vi "SLM_Holo to BMP.vi"(1 "path to BMP file":path=path "C:/Users/science/Desktop/Filippo The 2nd/LabVIEW/Holos/SLMA/HG_2_2.bmp", 2 "Holo":u32[][](array[numeric])) -> ()   [LabVIEW 2024]
uses:
  <vilib>/Utility/miscctls.llb/LVBoundsTypeDef.ctl
panel:
  in  "Array":u32[](array[numeric])=[1, 2, 3, 4, 5, 6, 7, 8, 9, 10, 11, 12, 13, 14, 15, 16, 17, 18, 19, 20, 21, 22, 23, 24, 25, 26, 27, 28, 29, 30, 31, 32, 33, 34, 35, 36, 37, 38, 39, 40, 41, 42, 43, 44, 45, 46, 47, 48, 49, 50, 51, 52, 53, 54, 55, 56, 57, 58, 59, 60, 61, 62, 63, 64, 65, 66, 67, 68, 69, 70, 71, 72, 73, 74, 75, 76, 77, 78, 79, 80, 81, 82, 83, 84, 85, 86, 87, 88, 89, 90, 91, 92, 93, 94, 95, 96, 97, 98, 99, 100, 101, 102, 103, 104, 105, 106, 107, 108, 109, 110, 111, 112, 113, 114, 115, 116, 117, 118, 119, 120, 121, 122, 123, 124, 125, 126, 127, 128, 129, 130, 131, 132, 133, 134, 135, 136, 137, 138, 139, 140, 141, 142, 143, 144, 145, 146, 147, 148, 149, 150, 151, 152, 153, 154, 155, 156, 157, 158, 159, 160, 161, 162, 163, 164, 165, 166, 167, 168, 169, 170, 171, 172, 173, 174, 175, 176, 177, 178, 179, 180, 181, 182, 183, 184, 185, 186, 187, 188, 189, 190, 191, 192, 193, 194, 195, 196, 197, 198, 199, 200, 201, 202, 203, 204, 205, 206, 207, 208, 209, 210, 211, 212, 213, 214, 215, 216, 217, 218, 219, 220, 221, 222, 223, 224, 225, 226, 227, 228, 229, 230, 231, 232, 233, 234, 235, 236, 237, 238, 239, 240, 241, 242, 243, 244, 245, 246, 247, 248, 249, 250, 251, 252, 253, 254, 255, 256]
  out "holo A":picture
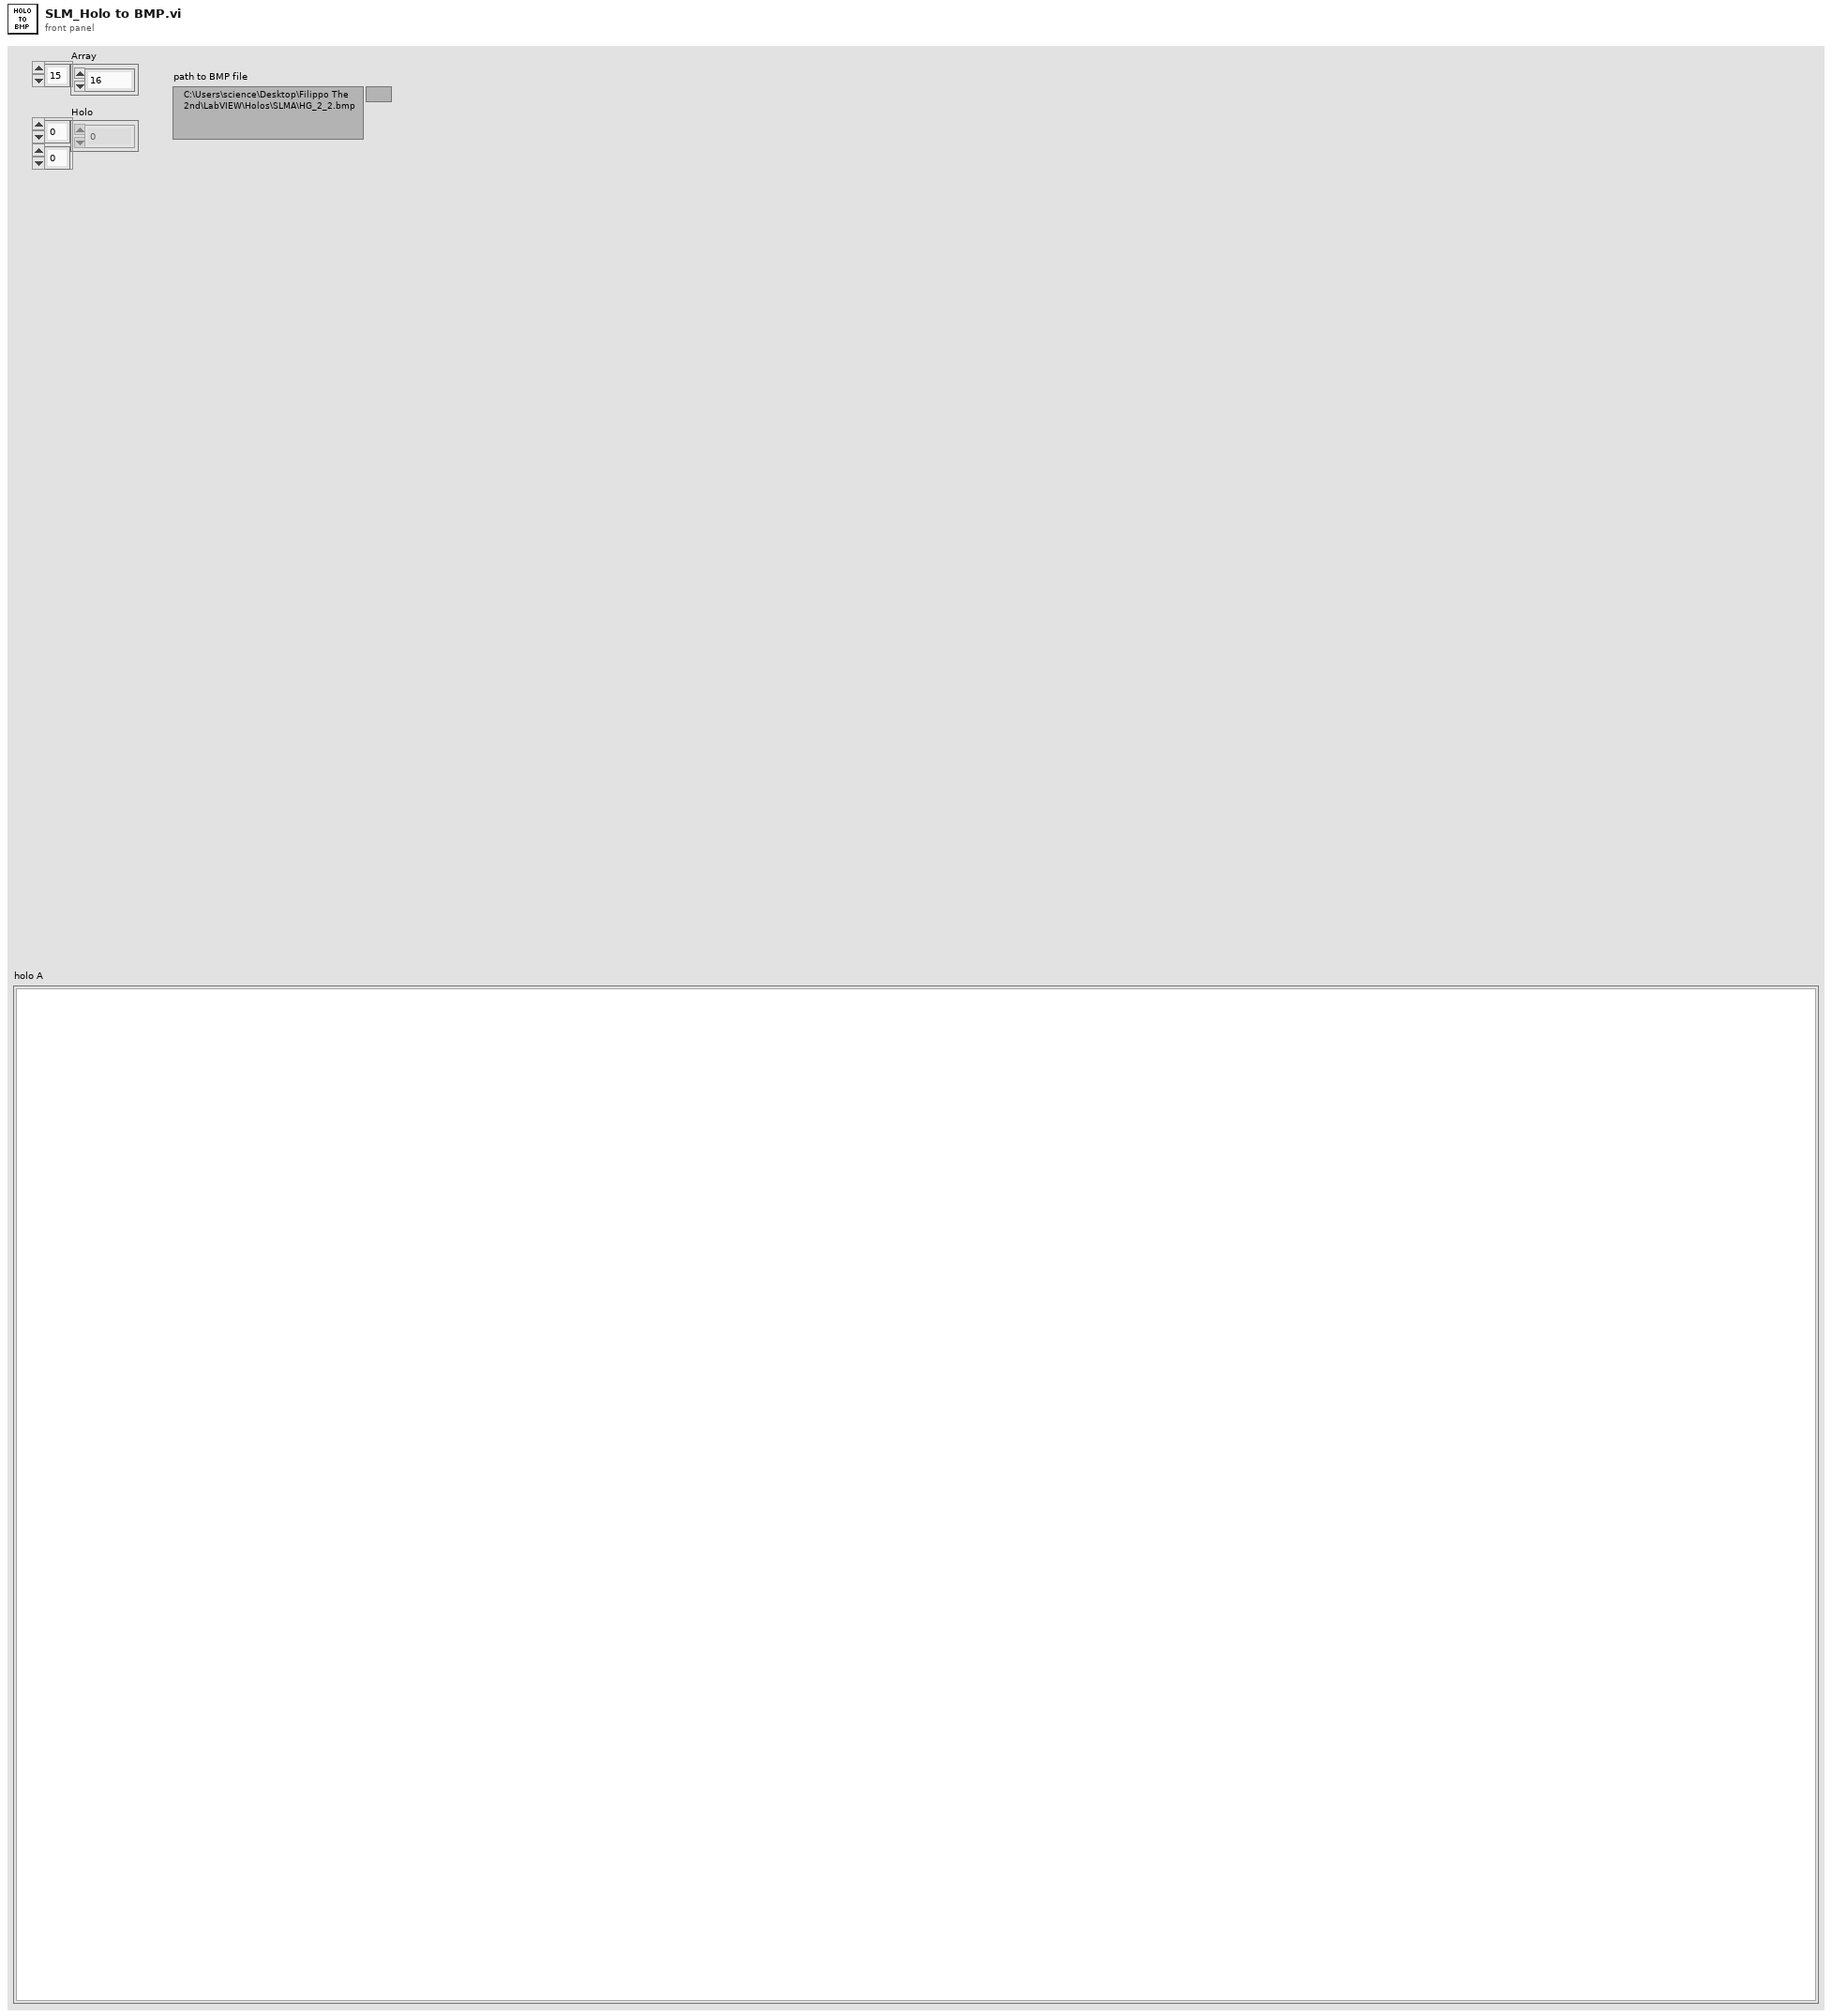
[diagram p1: front panel]
types:
  T1 = typedef "LVBoundsTypeDef.ctl" = cluster{"Width":u32, "Height":u32}
  T2 = cluster{"left":i16, "top":i16, "right":i16, "bottom":i16}
  T3 = typedef "imagedata.ctl" = cluster{"image type":i32, "image depth":i32, "image":u8[], "mask":u8[], "colors":u32[], "Rectangle":cluster{"left":i16, "top":i16, "right":i16, "bottom":i16}}
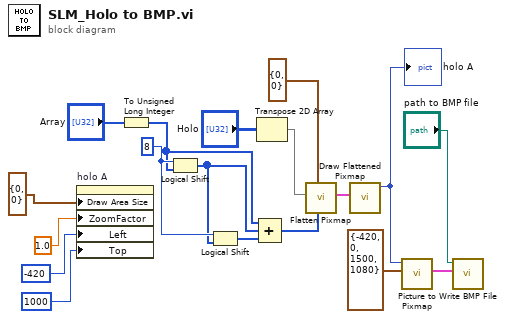
[diagram p0: block diagram]
diagram:
  w15 = i16 8 ("y")
  n1 = property on="holo A" class="Pict"("Draw Area Size"=T1 {"Width"=0, "Height"=0}, "ZoomFactor"=sgl 1.0 ("Zoom Factor"), "Left"=i16 -420 ("Origin:Left"), "Top"=1000 ("Position:Top")) -> ()  [unwired: 2 in, 2 out]
  n2 = To Unsigned Long Integer(number="Array") -> (unsigned 32bit integer=w14:u32[])
  n3 = Logical Shift(y=w15, x=w14) -> (x << y=w13:u32[])
  n4 = Logical Shift(y=w15, x=w13) -> (x << y=w16:u32[])
  n5 = Transpose 2D Array(2D array="Holo") -> (transposed array=w9:u32[][])
  n6 = Compound Arithmetic op=ADD(w14, w13, w16) -> (w12:u32[])
  n7 = call <vilib>:"Flatten Pixmap.vi"("colors"=w12, "top left"=cluster{"x":i16, "y":i16} {"x"=0, "y"=0}, "8-bit pixmap"=w9) -> ("image data"=w11:T3)  [unwired: 8 in]
  n8 = call <vilib>:"Draw Flattened Pixmap.vi"("image data"=w11) -> ("new picture"=w7:picture)  [unwired: 8 in]
  "holo A" <- w7
  n9 = call <vilib>:"Picture to Pixmap.vi"("rect"=T2 {"left"=-420, "top"=0, "right"=1500, "bottom"=1080}, "picture"=w7) -> ("image data"=w6:T3)  [unwired: 8 in, 1 out]
  n10 = call <vilib>:"Write BMP File.vi"("image data"=w6, "path to BMP file"="path to BMP file") -> ()  [unwired: 8 in, 2 out]
